vi "SDG60ConfModulationDSBAMnoch1.vi"(0 "VISA resource name":refnum<visa-resource-name>="USB0::0xF4EC::0x1101::SDG6XEBC5R0119::INSTR", 2 "Channel (1:Channel 1)":i32(ring)=1 items=["Channel 1"=1, "Channel 2"=2], 11 "error in (no error)":errorcluster) -> (4 "VISA resource name out":refnum<visa-resource-name>, 15 "error out":errorcluster)   [LabVIEW 2018]
doc: "Selects the waveform shape, frequency, amplitude, offset, and phase for standard waveforms (including Sine, Square, Ramp, Pulse, DC and Arb).\n\nNotes: \nTo configure other parameters for pulse waveforms please run the Configure Pulse VI. \nTo configure noise waveform please run the Configure Noise VI.\nTo configure other parameters for arbitrary waveforms please run the Create Arbitrary Waveform. \nTo configure PRBS waveform please run the Configure PRBS Waveform VI."
panel:
  in  "Frequency (1 Hz)":dbl=1000.0 format="%#_16g"
  in  "Mod wave shape (0:Sine)":u16(ring) items=["Sine", "Square", "Triangle", "Up Ramp", "Down Ramp", "Noise", "Arb"]
  in  "Internal/External (0: INT)":u16(ring) items=["Internal", "External"]
  # "DSBAM-Double-sideband amplitude modulation"
  # "Modulation will be turned on, as needed to be on to change\nsettings"
  # "Will reduce carrier frequency, leaving sidebands"
  # "Can set WFM then use this vi. No need to use CARR commands\nModulation can't be done on noise, DC (Not testing IQ as has trials)\nSet modulaton after setting up carrier WFM."
  # "Range: 0.001Hz-1 MHz\n11 digit precision"
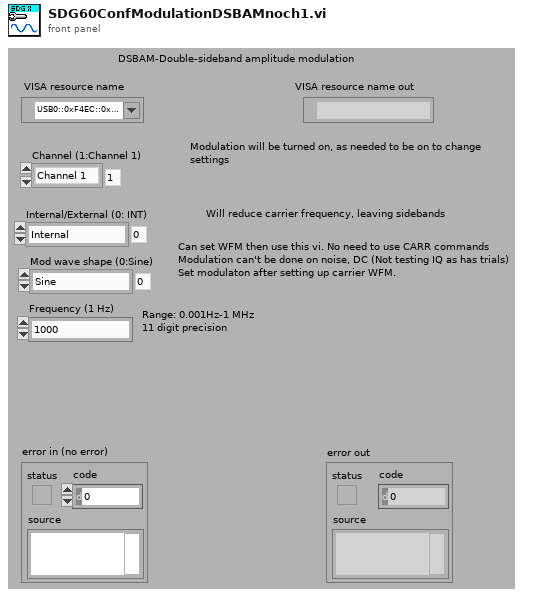
[diagram p1: front panel]
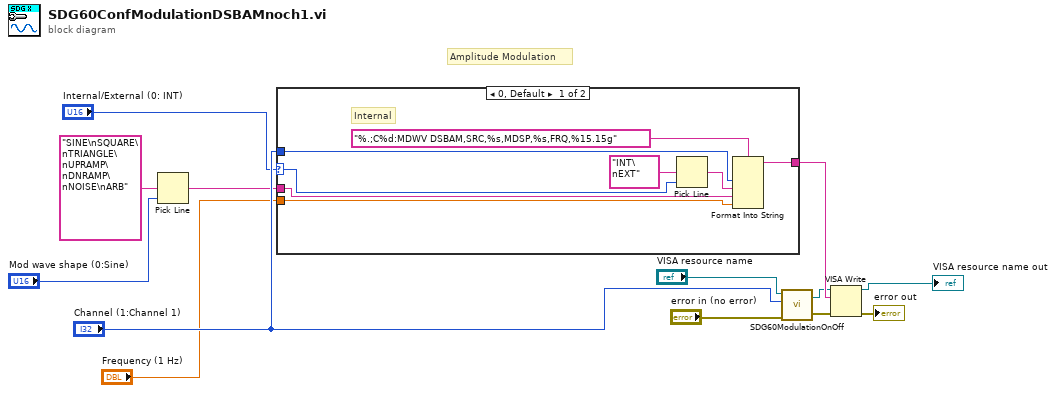
[diagram p0: block diagram]
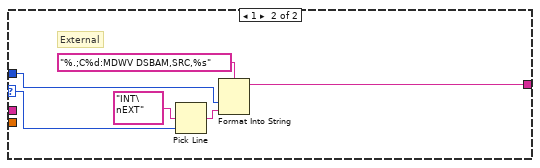
[diagram p2: hidden frame]
diagram:
  # "Amplitude Modulation"
  n1 = Pick Line(multi-line string="SINE\nSQUARE\nTRIANGLE\nUPRAMP\nDNRAMP\nNOISE\nARB", line index="Mod wave shape (0:Sine)") -> (output string=w2:string)  [unwired: 1 in]
  n2 = case shown="0, Default" "Internal/External (0: INT)" {
    selector: "Internal/External (0: INT)" -> [w18 w24]
    tunnel: [w20 w26] -> w13
    tunnel: "Channel (1:Channel 1)" -> [w19 w25]
    tunnel: w2 -> [w15 _]
    tunnel: "Frequency (1 Hz)" -> [w14 _]
    frame 0, Default {
      # "Internal"
      n3 = Pick Line(multi-line string="INT\nEXT", line index=w18) -> (output string=w16:string)  [unwired: 1 in]
      n4 = Format Into String(format string="%.;C%d:MDWV DSBAM,SRC,%s,MDSP,%s,FRQ,%15.15g", w19, w16, w15, w14) -> (resulting string=w20:string)  [unwired: 2 in, 1 out]
    }
    frame 1 {
      # "External"
      n5 = Pick Line(multi-line string="INT\nEXT", line index=w24) -> (output string=w22:string)  [unwired: 1 in]
      n6 = Format Into String(format string="%.;C%d:MDWV DSBAM,SRC,%s", w25, w22) -> (resulting string=w26:string)  [unwired: 2 in, 1 out]
    }
  }
  n7 = call "SDG60ModulationOnOff.vi"("error in (no error)"="error in (no error)", "Channel (1: Channel1)"="Channel (1:Channel 1)", "VISA resource name"="VISA resource name") -> ("error out"=w9:errorcluster, "VISA resource name out"=w7:refnum<visa-resource-name>)  [unwired: 1 in]
  n8 = VISA Write(VISA resource name=w7, write buffer=w13, error in (no error)=w9) -> (VISA resource name out=→"VISA resource name out":refnum<visa-resource-name>, error out=→"error out":errorcluster)  [unwired: 1 out]
